vi "SS2 Live_(Sub)Image Size.vi"(6 "Image Binning Options":T1={"Use Image Binning"=FALSE, "X Bin"=1, "Y Bin"=1} {"Y Bin" min=1; "X Bin" min=1}, 8 "Image Information":T2, 9 "# Pixel Y in":i32, 11 "# Pixel X in":i32) -> (1 "# Pixel Y out":i32, 3 "# Pixel X out":i32)   [LabVIEW 2019]
uses:
  SS2 Live_Image ROI Information.ctl
  Phasor/Image Binning Options.ctl
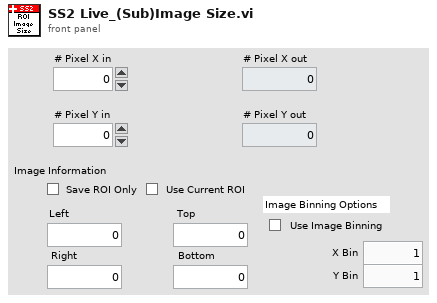
[diagram p1: front panel]
types:
  T1 = typedef "Image Binning Options.ctl" = cluster{"Use Image Binning":bool, "X Bin":i32, "Y Bin":i32}
  T2 = typedef "SS2 Live_Image ROI Information.ctl" = cluster{"Save ROI Only":bool, "Left":u16, "Top":u16, "Right":u16, "Bottom":u16, "Use Current ROI":bool}
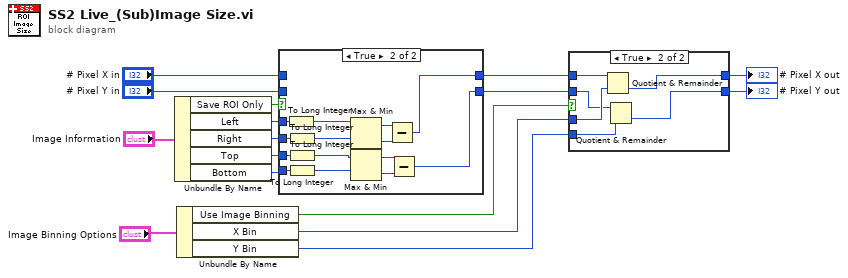
[diagram p0: block diagram]
diagram:
  n1 = Unbundle By Name("Image Information") -> ("Save ROI Only"=w14:bool, "Left"=w12:u16, "Right"=w10:u16, "Top"=w11:u16, "Bottom"=w9:u16)
  n2 = Unbundle By Name("Image Binning Options") -> ("Use Image Binning"=w7:bool, "X Bin"=w6:i32, "Y Bin"=w5:i32)
  n3 = case shown="True" w14 {
    tunnel: "# Pixel X in" -> [w18 _]
    tunnel: "# Pixel Y in" -> [w17 _]
    tunnel: [w18 w26] -> w4
    tunnel: [w17 w23] -> w3
    tunnel: w12 -> [_ w32]
    tunnel: w11 -> [_ w31]
    tunnel: w10 -> [_ w29]
    tunnel: w9 -> [_ w30]
    frame False {
    }
    frame True {
      n4 = To Long Integer(number=w32) -> (32bit integer=w22:i32)
      n5 = To Long Integer(number=w29) -> (32bit integer=w20:i32)
      n6 = To Long Integer(number=w31) -> (32bit integer=w19:i32)
      n7 = To Long Integer(number=w30) -> (32bit integer=w21:i32)
      n8 = Max & Min(x=w22, y=w20) -> (max(x,y)=w28:i32, min(x,y)=w27:i32)
      n9 = Max & Min(x=w19, y=w21) -> (max(x,y)=w25:i32, min(x,y)=w24:i32)
      n10 = Subtract(x=w28, y=w27) -> (x-y=w26:i32)
      n11 = Subtract(x=w25, y=w24) -> (x-y=w23:i32)
    }
  }
  n12 = case shown="True" w7 {
    tunnel: w6 -> [_ w39]
    tunnel: w5 -> [_ w36]
    tunnel: w4 -> [w34 w40]
    tunnel: w3 -> [w33 w37]
    tunnel: [w34 w38] -> w2
    tunnel: [w33 w35] -> w1
    frame False {
    }
    frame True {
      n13 = Quotient & Remainder(x=w40, y=w39) -> (floor(x/y)=w38:i32)  [unwired: 1 out]
      n14 = Quotient & Remainder(x=w37, y=w36) -> (floor(x/y)=w35:i32)  [unwired: 1 out]
    }
  }
  "# Pixel X out" <- w2
  "# Pixel Y out" <- w1
